vi "command_editor.vi"(1 "s/div":dbl=0.00025 format="%#_6p", 2 "Control":T1(array[cluster])=[{"Device"=10, "Operation"=0, "Command/byte count"="OUTP:LOAD INF\nAPPL:SIN 1000,10,0"}, {"Device"=1, "Operation"=0, "Command/byte count"="HEAD OFF\nDAT:SOU CH1\nDAT:ENC ASCI\nDAT:WID 1\nDAT:STAR 1\nDAT:STOP 2500\nCH1:SCA 1\nHOR:MAI:SCA 250E-6\nCURV?"}, {"Device"=1, "Operation"=1, "Command/byte count"="15000"}] {"Operation" items=["write", "read"]; "Device" items=["DSO"=1, "AWG"=10]}) -> (0 "output array":T1(array[cluster]))   [LabVIEW 2022 SP3]
panel:
  out "output cluster":T2
  out "Engineering string":string
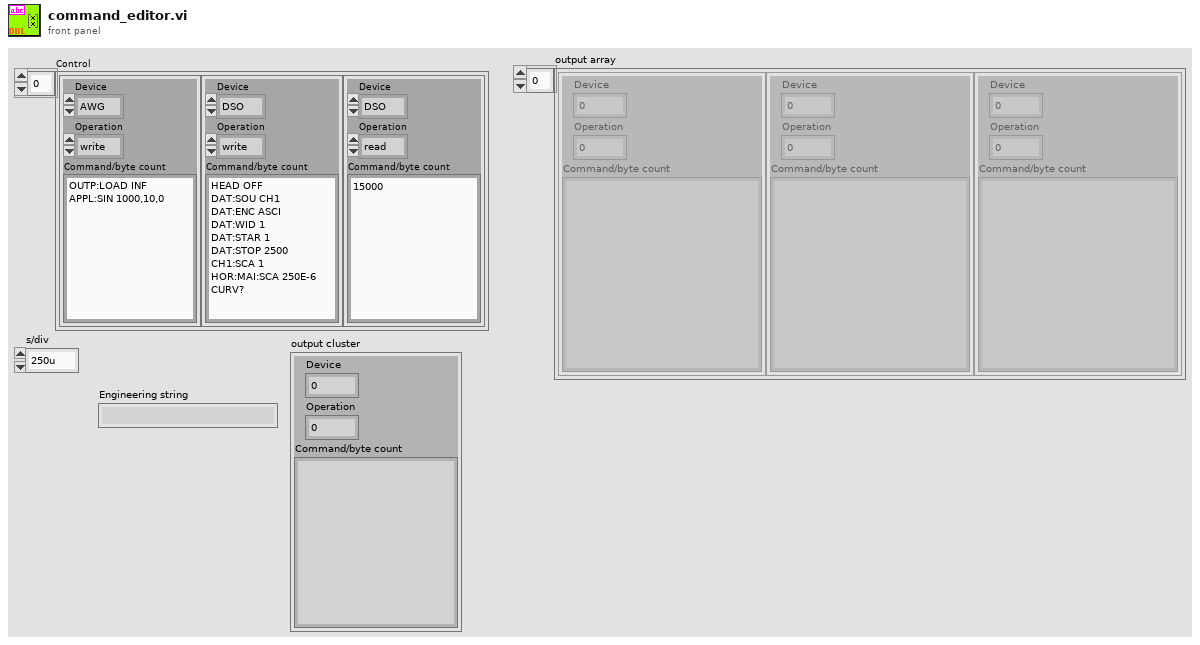
[diagram p1: front panel]
types:
  T1 = cluster{"Device":u16, "Operation":u16, "Command/byte count":string}[]
  T2 = cluster{"Device":u16, "Operation":u16, "Command/byte count":string}
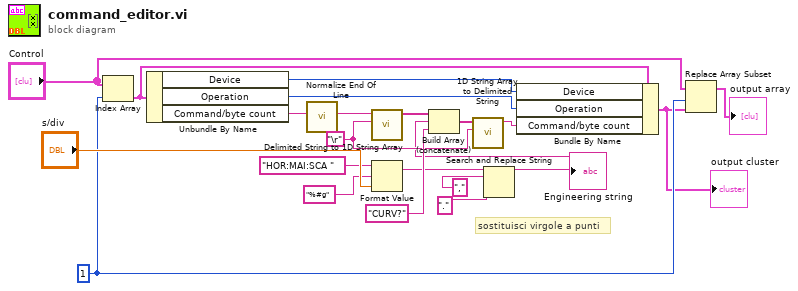
[diagram p0: block diagram]
diagram:
  w10 = "\r"
  w7 = 1 ("index")
  # "sostituisci virgole a punti"
  n1 = Index Array(array="Control", index=w7) -> (element=w14:T2)
  n2 = Unbundle By Name(w14) -> ("Device"=w13:u16, "Operation"=w12:u16, "Command/byte count"=w21:string)
  n3 = call <vilib>:"Normalize End Of Line.vi"("string in"=w21) -> ("string out"=w20:string)  [unwired: 7 in]
  n4 = call <vilib>:"Delimited String to 1D String Array.vi"("delimiter"=w10, "delimited string"=w20) -> ("string array"=w19:string[])  [unwired: 9 in]
  n5 = Format Value(string ("")="HOR:MAI:SCA " ("String"), format string="%#g", value (0)="s/div") -> (output string=w2:string)
  n6 = Search and Replace String(input string=w2, search string=",", replace string="." ("replace string (\"\")")) -> (result string=w1:string)  [unwired: 5 in, 3 out]
  "Engineering string" <- w1
  n7 = Build Array (concatenate)(w19, w1, "CURV?" ("String")) -> (w11:string[])
  n8 = call <vilib>:"1D String Array to Delimited String.vi"("delimiter"=w10, "string array"=w11) -> ("delimited string"=w9:string)  [unwired: 9 in]
  n9 = Bundle By Name(cluster=w14, "Device"=w13, "Operation"=w12, "Command/byte count"=w9) -> (w6:T2)
  "output cluster" <- w6
  n10 = Replace Array Subset(array="Control", new element=w6, index=w7) -> (→"output array":T1)
